vi "E3631A_Config.vi"(0 "VISA resource name":refnum<visa-resource-name>, 1 "CH-1 Voltage":dbl format="%.3g", 2 "CH-1 Current Limit":dbl=0.01 format="%.3g", 3 "CH-2 Voltage":dbl format="%.3g", 4 "CH-2 Current Limit":dbl=0.01 format="%.3g", 5 "error in (no error)":errorcluster, 6 "Reset":bool, 8 "ID Query":bool, 9 "Configure CH-1 ?":bool=TRUE, 11 "Configure Ch-2 ?":bool=TRUE, 12 "Enable Output":bool=TRUE) -> (16 "status":bool, 19 "error out":errorcluster)   [LabVIEW 2019]
uses:
  <userlib>/_TI-LA/Instr Drivers/Power Supply/E363x/Driver/Base/Agilent E363X Series.lvlib
panel:
  in  "Tab Control":T1(tab)
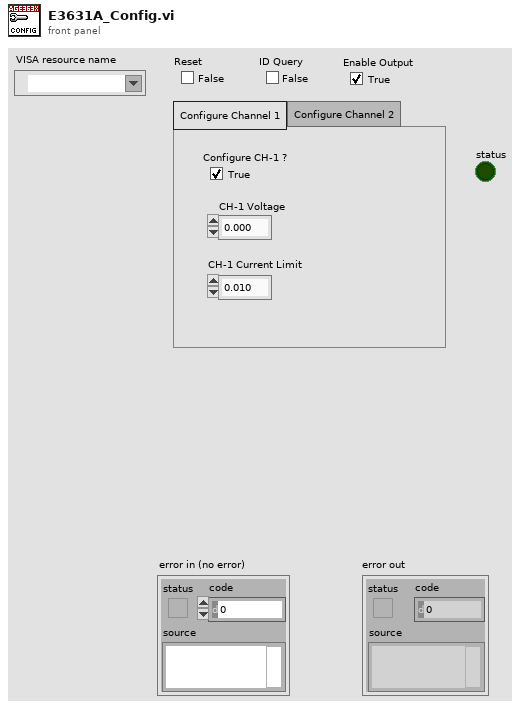
[diagram p1: front panel]
types:
  T1 = enum32{"Configure Channel 1", "Configure Channel 2"}
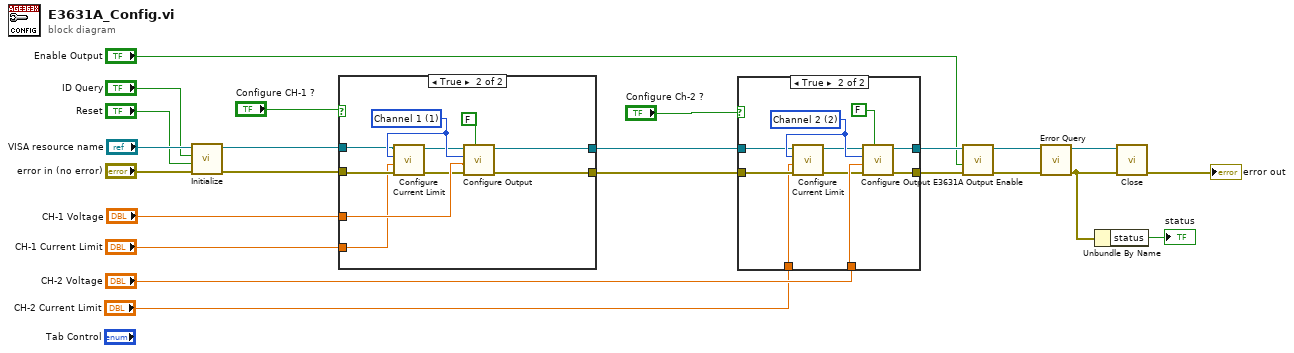
[diagram p0: block diagram]
diagram:
  n1 = call <userlib>:"Initialize.vi"("error in (no error)"="error in (no error)", "Reset? (T: Yes)"="Reset", "ID Query? (T: Yes)"="ID Query", "VISA resource name"="VISA resource name") -> ("error out"=w20:errorcluster, "VISA resource name out"=w21:refnum<visa-resource-name>)  [unwired: 6 in]
  n2 = case shown="True" "Configure CH-1 ?" {
    tunnel: w21 -> [w25 w33]
    tunnel: w20 -> [w24 w30]
    tunnel: "CH-1 Voltage" -> [_ w35]
    tunnel: "CH-1 Current Limit" -> [_ w29]
    tunnel: [w25 w27] -> w13
    tunnel: [w24 w28] -> w12
    frame False {
    }
    frame True {
      w34 = 1 items=["Channel 1"=1, "Channel 2"=2, "Channel 3"=3] ("Channel (1: Channel 1)")
      n3 = call <userlib>:"Configure Current Limit.vi"("error in (no error)"=w30, "Current Limit (0.0 A)"=w29, "Channel (1: Channel 1)"=w34, "VISA resource name"=w33) -> ("error out"=w31:errorcluster, "VISA resource name out"=w32:refnum<visa-resource-name>)  [unwired: 6 in]
      n4 = call <userlib>:"Configure Output.vi"("Enable Output (T: Enable)"=FALSE, "error in (no error)"=w31, "Voltage Level (0.0 V)"=w35, "Channel (1: Channel 1)"=w34, "VISA resource name"=w32) -> ("error out"=w28:errorcluster, "VISA resource name out"=w27:refnum<visa-resource-name>)  [unwired: 5 in]
    }
  }
  n5 = case shown="True" "Configure Ch-2 ?" {
    tunnel: w13 -> [w37 w45]
    tunnel: w12 -> [w36 w42]
    tunnel: "CH-2 Voltage" -> [_ w47]
    tunnel: "CH-2 Current Limit" -> [_ w41]
    tunnel: [w37 w39] -> w6
    tunnel: [w36 w40] -> w5
    frame False {
    }
    frame True {
      w46 = 2 items=["Channel 1"=1, "Channel 2"=2, "Channel 3"=3] ("Channel (1: Channel 1)")
      n6 = call <userlib>:"Configure Current Limit.vi"("error in (no error)"=w42, "Current Limit (0.0 A)"=w41, "Channel (1: Channel 1)"=w46, "VISA resource name"=w45) -> ("error out"=w43:errorcluster, "VISA resource name out"=w44:refnum<visa-resource-name>)  [unwired: 6 in]
      n7 = call <userlib>:"Configure Output.vi"("Enable Output (T: Enable)"=FALSE, "error in (no error)"=w43, "Voltage Level (0.0 V)"=w47, "Channel (1: Channel 1)"=w46, "VISA resource name"=w44) -> ("error out"=w40:errorcluster, "VISA resource name out"=w39:refnum<visa-resource-name>)  [unwired: 5 in]
    }
  }
  n8 = call "E3631A Output Enable.vi"("error in (no error)"=w5, "Output ?"="Enable Output", "VISA session"=w6) -> ("error out"=w2:errorcluster, "VISA resource name Out"=w3:refnum<visa-resource-name>)  [unwired: 7 in]
  n9 = call <userlib>:"Error Query.vi"("error in (no error)"=w2, "VISA resource name"=w3) -> ("error out"=w1:errorcluster, "VISA resource name out"=w8:refnum<visa-resource-name>)  [unwired: 6 in, 2 out]
  n10 = Unbundle By Name(w1) -> ("status"=→"status":bool)
  n11 = call <userlib>:"Close.vi"("error in (no error)"=w1, "VISA resource name"=w8) -> ("error out"=→"error out":errorcluster)  [unwired: 9 in]
